vi "Default Instrument Setup.vi"(8 "error in (no error)":errorcluster, 11 "VISA resource name":refnum<visa-resource-name>) -> (0 "error out":errorcluster, 3 "VISA resource name out":refnum<visa-resource-name>)   [LabVIEW 2020, in "Agilent E363X Series.lvlib"]
doc: "This Utility VI sends a default command string to the instrument whenever a new VISA session is opened, or the instrument is reset. This VI is intended to be used as a subVI for the <B>Initialize</B> and <B>Reset</B> VI's. Altering this VI could cause these two VI's to operate incorrectly."
uses:
  Agilent E363X Series.lvlib
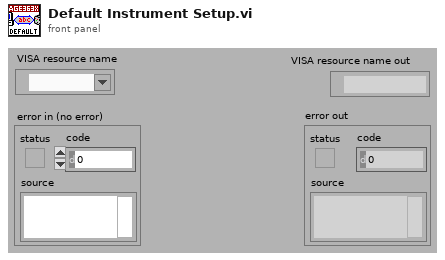
[diagram p1: front panel]
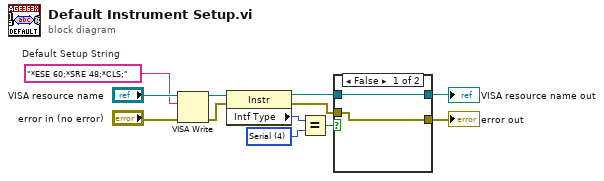
[diagram p0: block diagram]
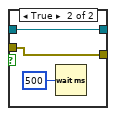
[diagram p2: hidden frame]
diagram:
  w5 = u16 4 items=["GPIB"=1, "VXI"=2, "GPIB-VXI"=3, "Serial"=4, "PXI"=5, "TCPIP"=6, "USB"=7] ("Interface Information:Interface Type")
  w10 = "*ESE 60;*SRE 48;*CLS;"  # Default Setup String
  n1 = VISA Write(VISA resource name="VISA resource name", write buffer=w10, error in (no error)="error in (no error)") -> (VISA resource name out=w8:refnum<visa-resource-name>, error out=w9:errorcluster)  [unwired: 1 out]
  n2 = property class="Instr"(reference=w8, error in=w9) -> (reference out=w4:refnum<visa-resource-name>, error out=w2:errorcluster, "Intf Type"=w6:u16)
  n3 = Equal?(x=w6, y=w5) -> (x = y?=w7:bool)
  n4 = case shown="False" w7 {
    tunnel: w4 -> [w14 w17]
    tunnel: [w14 w17] -> w3
    tunnel: w2 -> [w13 w16]
    tunnel: [w13 w16] -> w1
    frame False {
    }
    frame True {
      n5 = Wait (ms)(milliseconds to wait=u32 500) -> ()  [unwired: 1 out]
    }
  }
  "error out" <- w1
  "VISA resource name out" <- w3
